vi "Code Point to UTF-8.vi"(10 "Code Point":string) -> (2 "UTF-8":string)   [LabVIEW 2020, in "TOML.lvlib"]
uses:
  TOML.lvlib
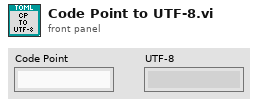
[diagram p1: front panel]
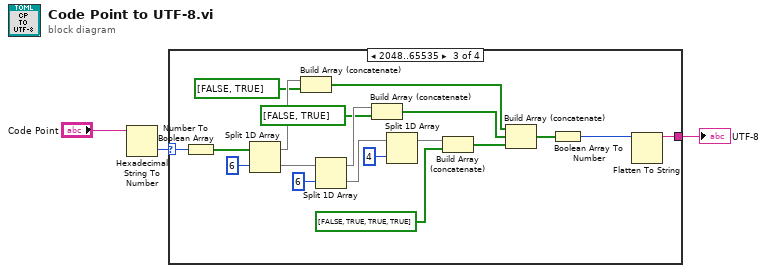
[diagram p0: block diagram]
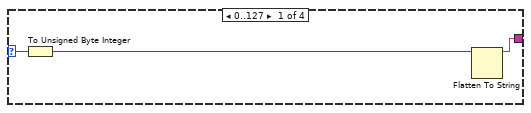
[diagram p2: hidden frame]
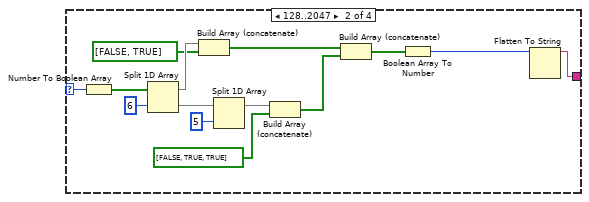
[diagram p3: hidden frame]
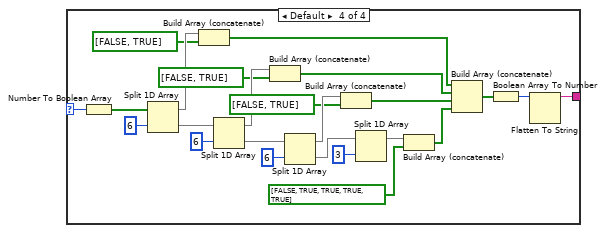
[diagram p4: hidden frame]
diagram:
  n1 = Hexadecimal String To Number(string="Code Point") -> (number=w1:u32)  [unwired: 2 in, 1 out]
  n2 = case shown="2048..65535" w1 {
    selector: w1 -> [w6 w20 w39 w63]
    tunnel: [w4 w8 w27 w51] -> w2
    frame 0..127 {
      n3 = To Unsigned Byte Integer(number=w6) -> (unsigned 8bit integer=w5:u8)
      n4 = Flatten To String(anything=w5) -> (data string=w4:string)  [unwired: 3 in, 2 out]
    }
    frame 128..2047 {
      n5 = Number To Boolean Array(number=w20) -> (Boolean array=w19:bool[])
      n6 = Split 1D Array(array=w19, index=6) -> (first subarray=w15:bool[], second subarray=w17:bool[])
      n7 = Build Array (concatenate)(w15, bool[] [FALSE, TRUE] ("element")) -> (w10:bool[])
      n8 = Split 1D Array(array=w17, index=5) -> (first subarray=w13:bool[])  [unwired: 1 out]
      n9 = Build Array (concatenate)(w13, bool[] [FALSE, TRUE, TRUE] ("element")) -> (w11:bool[])
      n10 = Build Array (concatenate)(w10, w11) -> (w7:bool[])
      n11 = Boolean Array To Number(Boolean array=w7) -> (number=w9:u16)
      n12 = Flatten To String(anything=w9) -> (data string=w8:string)  [unwired: 3 in, 2 out]
    }
    frame 2048..65535 {
      n13 = Number To Boolean Array(number=w39) -> (Boolean array=w38:bool[])
      n14 = Split 1D Array(array=w38, index=6) -> (first subarray=w34:bool[], second subarray=w36:bool[])
      n15 = Build Array (concatenate)(w34, bool[] [FALSE, TRUE] ("element")) -> (w29:bool[])
      n16 = Split 1D Array(array=w36, index=6) -> (first subarray=w32:bool[], second subarray=w23:bool[])
      n17 = Build Array (concatenate)(w32, bool[] [FALSE, TRUE] ("element")) -> (w30:bool[])
      n18 = Split 1D Array(array=w23, index=4) -> (first subarray=w22:bool[])  [unwired: 1 out]
      n19 = Build Array (concatenate)(w22, bool[] [FALSE, TRUE, TRUE, TRUE] ("element")) -> (w21:bool[])
      n20 = Build Array (concatenate)(w29, w30, w21) -> (w26:bool[])
      n21 = Boolean Array To Number(Boolean array=w26) -> (number=w28:u32)
      n22 = Flatten To String(anything=w28) -> (data string=w27:string)  [unwired: 3 in, 2 out]
    }
    frame Default {
      n23 = Number To Boolean Array(number=w63) -> (Boolean array=w62:bool[])
      n24 = Split 1D Array(array=w62, index=6) -> (first subarray=w58:bool[], second subarray=w60:bool[])
      n25 = Build Array (concatenate)(w58, bool[] [FALSE, TRUE] ("element")) -> (w53:bool[])
      n26 = Split 1D Array(array=w60, index=6) -> (first subarray=w56:bool[], second subarray=w48:bool[])
      n27 = Build Array (concatenate)(w56, bool[] [FALSE, TRUE] ("element")) -> (w54:bool[])
      n28 = Split 1D Array(array=w48, index=6) -> (first subarray=w47:bool[], second subarray=w42:bool[])
      n29 = Build Array (concatenate)(w47, bool[] [FALSE, TRUE] ("element")) -> (w46:bool[])
      n30 = Split 1D Array(array=w42, index=3) -> (first subarray=w40:bool[])  [unwired: 1 out]
      n31 = Build Array (concatenate)(w40, bool[] [FALSE, TRUE, TRUE, TRUE, TRUE] ("element")) -> (w41:bool[])
      n32 = Build Array (concatenate)(w53, w54, w46, w41) -> (w50:bool[])
      n33 = Boolean Array To Number(Boolean array=w50) -> (number=w52:u32)
      n34 = Flatten To String(anything=w52) -> (data string=w51:string)  [unwired: 3 in, 2 out]
    }
  }
  "UTF-8" <- w2
